vi "WPI_I2CERRSensorMismatch.vi"(9 "Read From Sensor":string, 10 "Expected":string) -> (0 "ERRSensorMismatch":errorcluster)   [LabVIEW 2017]
doc: "This software is licensed. Open the labview\\readme\\WPI Robotics Library Open Source License.txt file for more information."
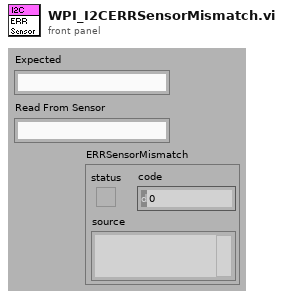
[diagram p1: front panel]
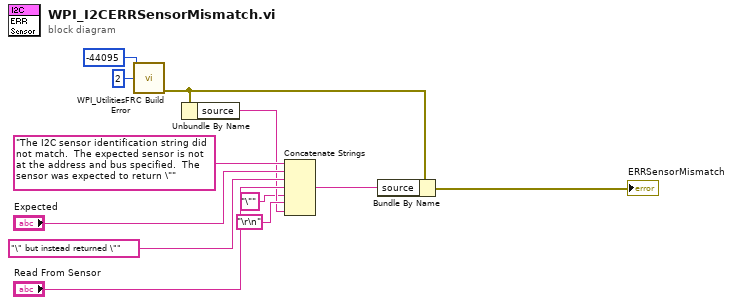
[diagram p0: block diagram]
diagram:
  n1 = call <vilib>:"WPI_UtilitiesFRC Build Error.vi"("error code"=-44095 ("code"), "chain levels to remove (1)"=2) -> ("error out"=w4:errorcluster)  [unwired: 3 in, 10 out]
  n2 = Unbundle By Name(w4) -> ("source"=w2:string)
  n3 = Concatenate Strings("The I2C sensor identification string did not match.  The expected sensor is not at the address and bus specified.  The sensor was expected to return \"", "Expected", "\" but instead returned \"", "Read From Sensor", "\"", "\r\n", w2) -> (w11:string)
  n4 = Bundle By Name(cluster=w4, "source"=w11) -> (→"ERRSensorMismatch":errorcluster)
